vi "MS_Stage_Control_counter.vi"() -> ()   [LabVIEW 2016]
uses:
  <vilib>/DAQmx/read.llb/DAQmx Read (Counter U32 1Chan 1Samp).vi
  Utility/Global Constants.vi
  Utility/Global_Laser.vi
  <vilib>/Utility/file.llb/Read From Spreadsheet File (DBL).vi
  <vilib>/DAQmx/miscellaneous.llb/DAQmx Fill In Error Info.vi
panel:
  out "x*y":u32
  out "Read out":sgl[][](array[numeric])
  out "Done?":bool
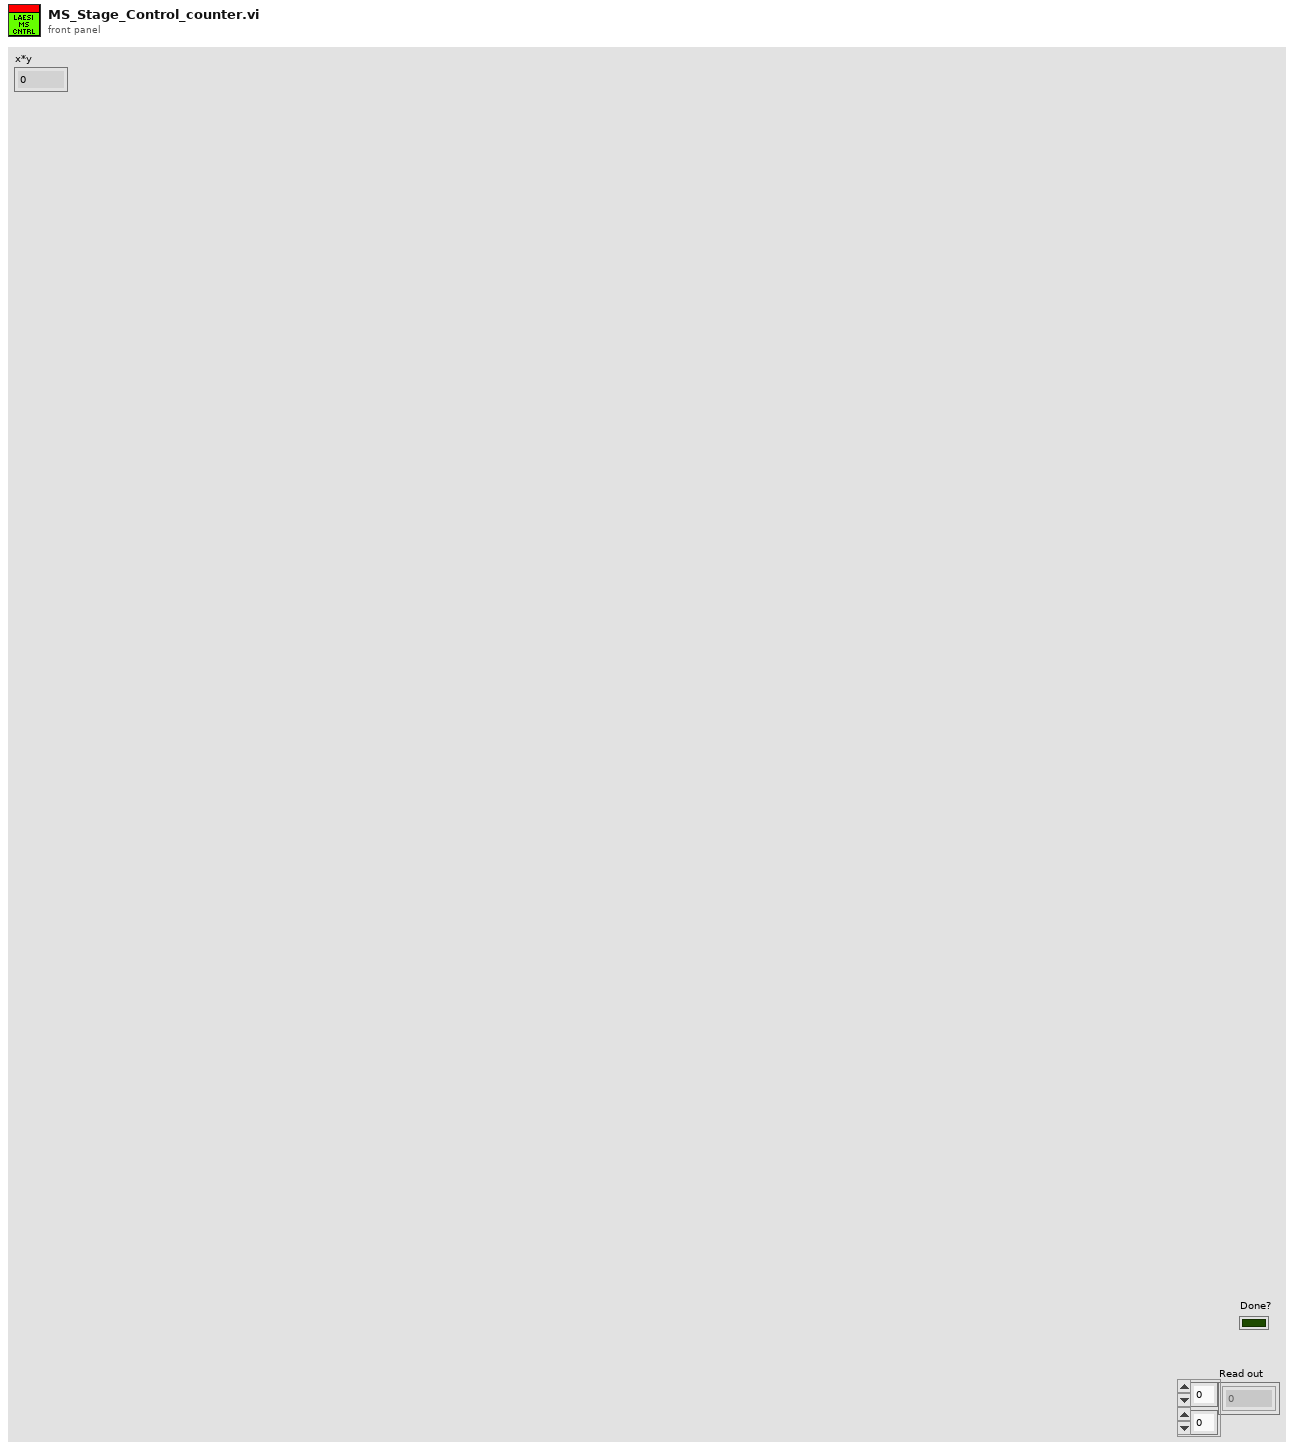
[diagram p1: front panel]
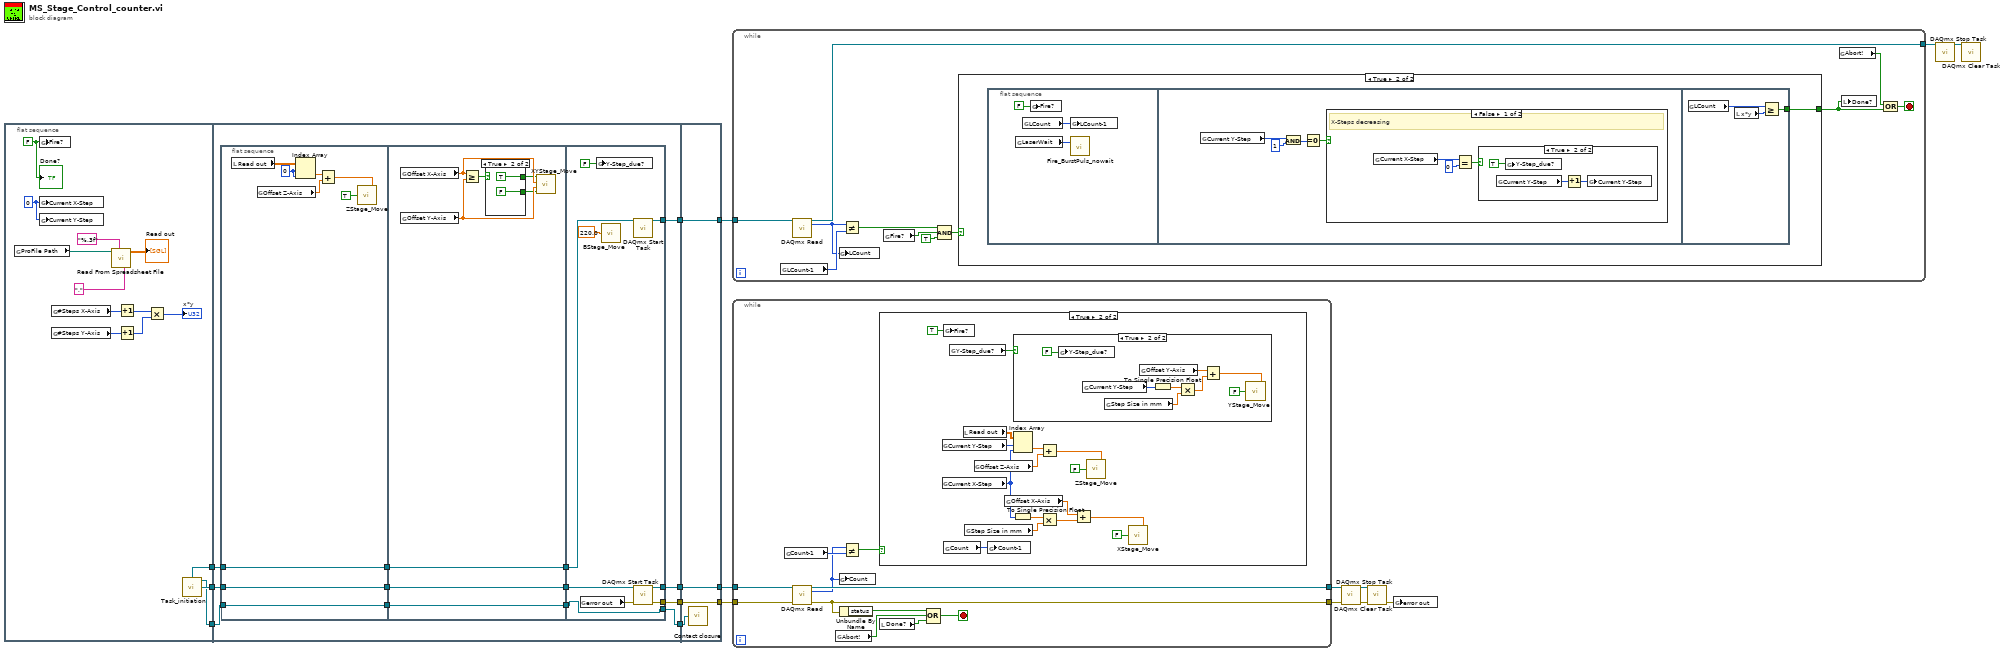
[diagram p0: block diagram]
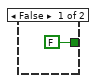
[diagram p4: hidden frame]
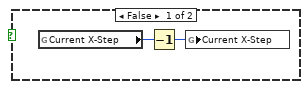
[diagram p5: hidden frame]
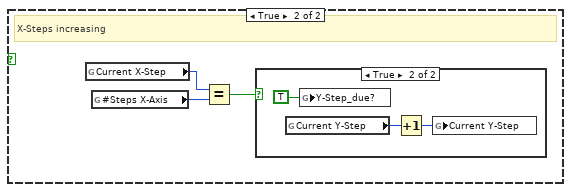
[diagram p6: hidden frame]
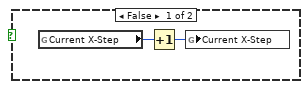
[diagram p7: hidden frame]
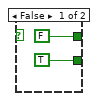
[diagram p8: hidden frame]
diagram:
  n1 = flat-sequence {
    tunnel: [w27] -> w17
    tunnel: [w26] -> w16
    tunnel: [w18] -> w1
    tunnel: w17 -> [w44]
    tunnel: [w41] -> w15
    tunnel: w16 -> [w40]
    tunnel: [w37] -> w14
    tunnel: [w36] -> w6
    tunnel: [w33] -> w2
    tunnel: w1 -> [w35]
    tunnel: [w78] -> w13
    tunnel: w14 -> [w78]
    tunnel: w15 -> [w77]
    tunnel: [w77] -> w7
    tunnel: w6 -> [w76]
    tunnel: [w76] -> w5
    tunnel: w2 -> [w75]
    frame #0 {
      w25 = FALSE
      w24 = 0 ("Current X-Step")
      n2 = global read "Global Constants.vi" "ProFile Path"() -> (w29:path)
      n3 = global write "Global_Laser.vi" "Fire?"(w25) -> ()
      n4 = global write "Global Constants.vi" "Current X-Step"(w24) -> ()
      n5 = global write "Global Constants.vi" "Current Y-Step"(w24) -> ()
      n6 = global read "Global Constants.vi" "#Steps X-Axis"() -> (w23:i32)
      n7 = global read "Global Constants.vi" "#Steps Y-Axis"() -> (w22:i32)
      n8 = call-poly <vilib>:"Read From Spreadsheet File.vi"("delimiter (\\t)"="," ("delimiter (\\t)"), "format (%.3f)"="%.3f", "file path (dialog if empty)"=w29) -> ("all rows"=→"Read out":dbl[][])  [unwired: 4 in, 4 out]
      n9 = Increment(x=w23) -> (x+1=w21:i32)
      n10 = Increment(x=w22) -> (x+1=w20:i32)
      n11 = Multiply(x=w21, y=w20) -> (x*y=→"x*y":i32)
      n12 = call "Task_initiation.vi"() -> ("task out\nlaser trigger"=w26:refnum<k21>, "task out\nedge count"=w27:refnum<k21>, "task out CC"=w18:refnum<k21>)
      "Done?" <- w25
    }
    frame #1 {
      n13 = flat-sequence {
        tunnel: w44 -> [w47]
        tunnel: [w47] -> w43
        tunnel: w40 -> [w46]
        tunnel: [w46] -> w38
        tunnel: w35 -> [w45]
        tunnel: [w45] -> w34
        tunnel: w43 -> [w56]
        tunnel: [w56] -> w42
        tunnel: [w55] -> w39
        tunnel: w38 -> [w55]
        tunnel: w34 -> [w54]
        tunnel: [w54] -> w32
        tunnel: w42 -> [w73]
        tunnel: [w72] -> w36
        tunnel: [w70] -> w41
        tunnel: w39 -> [w69]
        tunnel: [w68] -> w37
        tunnel: [w66] -> w33
        tunnel: w32 -> [w66]
        frame #0 {
          w52 = 0 ("index (row)")
          n14 = local read "Read out"() -> (w51:sgl[][])
          n15 = global read "Global Constants.vi" "Offset Z-Axis"() -> (w53:sgl)
          n16 = Index Array(array=w51, index (row)=w52, index (col)=w52) -> (element=w50:sgl)
          n17 = Add(x=w50, y=w53) -> (x+y=w49:sgl)
          n18 = call "ZStage_Move.vi"("Position"=w49, "Z_Wait"=TRUE) -> ()
        }
        frame #1 {
          n19 = global read "Global Constants.vi" "Offset X-Axis"() -> (w61:sgl)
          n20 = global read "Global Constants.vi" "Offset Y-Axis"() -> (w60:sgl)
          n21 = Greater Or Equal?(x=w61, y=w60) -> (x >= y?=w59:bool)
          n22 = case shown="True" w59 {
            tunnel: [FALSE TRUE] -> w58
            tunnel: [TRUE FALSE] -> w57
            frame False {
            }
            frame True {
            }
          }
          n23 = call "XYStage_Move.vi"("Y_Wait"=w57, "Position Y"=w60, "Position X"=w61, "X_Wait"=w58) -> ()
        }
        frame #2 {
          n24 = global read "Global Constants.vi" "error out"() -> (w71:errorcluster)
          n25 = global write "Global Constants.vi" "Y-Step_due?"(FALSE ("Y-Step_due?")) -> ()
          n26 = call "BStage_Move.vi"("Position"=sgl 220.0) -> ()
          n27 = call <vilib>:"DAQmx Start Task.vi"("task/channels in"=w69) -> ("task out"=w68:refnum<k21>)  [unwired: 13 in, 1 out]
          n28 = call <vilib>:"DAQmx Start Task.vi"("task/channels in"=w73, "error in"=w71) -> ("task out"=w72:refnum<k21>, "error out"=w70:errorcluster)  [unwired: 12 in]
        }
      }
    }
    frame #2 {
      n29 = call "Contact closure.vi"("Task In CC"=w75) -> ()
    }
  }
  n30 = while {
    tunnel: w13 -> [w87]
    tunnel: [w86] -> w12
    stop <- w88 stop-if-true
    n31 = global read "Global_Laser.vi" "LCount-1"() -> (w84:u32)
    n32 = call-poly <vilib>:"DAQmx Read.vi"("task/channels in"=w87) -> ("task out"=w86:refnum<k21>, "data"=w83:u32)  [unwired: 12 in, 1 out]
    n33 = global write "Global_Laser.vi" "LCount"(w83) -> ()
    n34 = Not Equal?(x=w83, y=w84) -> (x != y?=w85:bool)
    n35 = global read "Global_Laser.vi" "Fire?"() -> (w82:bool)
    n36 = Compound Arithmetic op=AND(w85, w82, TRUE ("value")) -> (w81:bool)
    n37 = case shown="True" w81 {
      tunnel: [FALSE w91] -> w79
      frame False {
      }
      frame True {
        n38 = flat-sequence {
          tunnel: [w115] -> w91
          frame #0 {
            n39 = global read "Global_Laser.vi" "LaserWait"() -> (w92:u32)
            n40 = global read "Global_Laser.vi" "LCount"() -> (w94:u32)
            n41 = global write "Global_Laser.vi" "Fire?"(FALSE) -> ()
            n42 = global write "Global_Laser.vi" "LCount-1"(w94) -> ()
            n43 = call "Fire_BurstPuls_nowait.vi"("milliseconds to wait"=w92) -> ()  [unwired: 1 in, 1 out]
          }
          frame #1 {
            n44 = global read "Global Constants.vi" "Current Y-Step"() -> (w96:i32)
            n45 = And(x=w96, y=1) -> (x .and. y?=w97:i32)
            n46 = Equal To 0?(x=w97) -> (x = 0?=w95:bool)
            n47 = case shown="False" w95 {
              frame False {
                # "X-Steps decreasing"
                n48 = global read "Global Constants.vi" "Current X-Step"() -> (w99:i32)
                n49 = Equal?(x=w99, y=0) -> (x = y?=w100:bool)
                n50 = case shown="True" w100 {
                  frame False {
                    n51 = global read "Global Constants.vi" "Current X-Step"() -> (w103:i32)
                    n52 = Decrement(x=w103) -> (x-1=w102:i32)
                    n53 = global write "Global Constants.vi" "Current X-Step"(w102) -> ()
                  }
                  frame True {
                    n54 = global read "Global Constants.vi" "Current Y-Step"() -> (w104:i32)
                    n55 = global write "Global Constants.vi" "Y-Step_due?"(TRUE) -> ()
                    n56 = Increment(x=w104) -> (x+1=w105:i32)
                    n57 = global write "Global Constants.vi" "Current Y-Step"(w105) -> ()
                  }
                }
              }
              frame True {
                # "X-Steps increasing"
                n58 = global read "Global Constants.vi" "Current X-Step"() -> (w108:i32)
                n59 = global read "Global Constants.vi" "#Steps X-Axis"() -> (w107:i32)
                n60 = Equal?(x=w108, y=w107) -> (x = y?=w109:bool)
                n61 = case shown="True" w109 {
                  frame False {
                    n62 = global read "Global Constants.vi" "Current X-Step"() -> (w111:i32)
                    n63 = Increment(x=w111) -> (x+1=w110:i32)
                    n64 = global write "Global Constants.vi" "Current X-Step"(w110) -> ()
                  }
                  frame True {
                    n65 = global read "Global Constants.vi" "Current Y-Step"() -> (w112:i32)
                    n66 = global write "Global Constants.vi" "Y-Step_due?"(TRUE) -> ()
                    n67 = Increment(x=w112) -> (x+1=w113:i32)
                    n68 = global write "Global Constants.vi" "Current Y-Step"(w113) -> ()
                  }
                }
              }
            }
          }
          frame #2 {
            n69 = global read "Global_Laser.vi" "LCount"() -> (w117:u32)
            n70 = local read "x*y"() -> (w116:u32)
            n71 = Greater Or Equal?(x=w117, y=w116) -> (x >= y?=w115:bool)
          }
        }
      }
    }
    n72 = global read "Global Constants.vi" "Abort!"() -> (w89:bool)
    n73 = local write "Done?"(w79) -> ()
    n74 = Compound Arithmetic op=OR(w89, w79) -> (w88:bool)
  }
  n75 = while {
    tunnel: w7 -> [w128]
    tunnel: w5 -> [w127]
    tunnel: [w125] -> w4
    tunnel: [w126] -> w3
    stop <- w120 stop-if-true
    n76 = global read "Global Constants.vi" "Count-1"() -> (w123:u32)
    n77 = call-poly <vilib>:"DAQmx Read.vi"("task/channels in"=w127, "error in"=w128) -> ("task out"=w125:refnum<k21>, "data"=w122:u32, "error out"=w126:errorcluster)  [unwired: 11 in]
    n78 = global read "Global Constants.vi" "Abort!"() -> (w119:bool)
    n79 = global write "Global Constants.vi" "Count"(w122) -> ()
    n80 = Unbundle By Name(w126) -> ("status"=w121:bool)
    n81 = Not Equal?(x=w122, y=w123) -> (x != y?=w124:bool)
    n82 = case shown="True" w124 {
      frame False {
      }
      frame True {
        n83 = global read "Global Constants.vi" "Current Y-Step"() -> (w132:i32)
        n84 = global read "Global Constants.vi" "Current X-Step"() -> (w131:i32)
        n85 = global write "Global_Laser.vi" "Fire?"(TRUE ("y")) -> ()
        n86 = global read "Global Constants.vi" "Count"() -> (w129:u32)
        n87 = global read "Global Constants.vi" "Y-Step_due?"() -> (w130:bool)
        n88 = local read "Read out"() -> (w141:sgl[][])
        n89 = global read "Global Constants.vi" "Step Size in mm"() -> (w142:sgl)
        n90 = global read "Global Constants.vi" "Offset Z-Axis"() -> (w133:sgl)
        n91 = global write "Global Constants.vi" "Count-1"(w129) -> ()
        n92 = global read "Global Constants.vi" "Offset X-Axis"() -> (w139:sgl)
        n93 = case shown="True" w130 {
          frame False {
          }
          frame True {
            n94 = global write "Global Constants.vi" "Y-Step_due?"(FALSE ("Y-Step_due?")) -> ()
            n95 = global read "Global Constants.vi" "Current Y-Step"() -> (w146:i32)
            n96 = global read "Global Constants.vi" "Step Size in mm"() -> (w148:sgl)
            n97 = global read "Global Constants.vi" "Offset Y-Axis"() -> (w149:sgl)
            n98 = To Single Precision Float(number=w146) -> (single precision float=w147:sgl)
            n99 = Multiply(x=w147, y=w148) -> (x*y=w150:sgl)
            n100 = Add(x=w149, y=w150) -> (x+y=w152:sgl)
            n101 = call "YStage_Move.vi"("Position"=w152, "Y_Wait"=FALSE ("bWait")) -> ()
          }
        }
        n102 = Index Array(array=w141, index (row)=w132, index (col)=w131) -> (element=w140:sgl)
        n103 = To Single Precision Float(number=w131) -> (single precision float=w143:sgl)
        n104 = Add(x=w140, y=w133) -> (x+y=w137:sgl)
        n105 = Multiply(x=w143, y=w142) -> (x*y=w138:sgl)
        n106 = Add(x=w139, y=w138) -> (x+y=w134:sgl)
        n107 = call "ZStage_Move.vi"("Position"=w137, "Z_Wait"=FALSE ("bWait")) -> ()
        n108 = call "XStage_Move.vi"("Position"=w134, "X_Wait"=FALSE ("bWait")) -> ()
      }
    }
    n109 = local read "Done?"() -> (w118:bool)
    n110 = Compound Arithmetic op=OR(w121, w119, w118) -> (w120:bool)
  }
  n111 = call <vilib>:"DAQmx Stop Task.vi"("task/channels in"=w4, "error in"=w3) -> ("task out"=w9:refnum<k21>, "error out"=w8:errorcluster)  [unwired: 12 in]
  n112 = call <vilib>:"DAQmx Clear Task.vi"("task in"=w9, "error in"=w8) -> ("error out"=w10:errorcluster)  [unwired: 13 in]
  n113 = global write "Global Constants.vi" "error out"(w10) -> ()
  n114 = call <vilib>:"DAQmx Stop Task.vi"("task/channels in"=w12) -> ("task out"=w11:refnum<k21>)  [unwired: 13 in, 1 out]
  n115 = call <vilib>:"DAQmx Clear Task.vi"("task in"=w11) -> ()  [unwired: 14 in, 1 out]
